vi "cloneAndCompare.vi"(9 "shapes":refnum<class "pShape.lvclass">[](array[class]), 10 "shapesCopy":refnum<class "pShape.lvclass">[](array[class])) -> ()   [LabVIEW 2017, in "PrototypePatternDemo.lvclass"]
uses:
  PrototypePatternDemo.lvclass
  Shape Class/pShape.lvclass
  ConsoleOut/Print Options.ctl
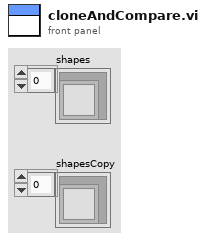
[diagram p1: front panel]
types:
  T1 = typedef "Print Options.ctl" = enum16{"Create", "Get Reference", "Print", "Print Header", "Close"}
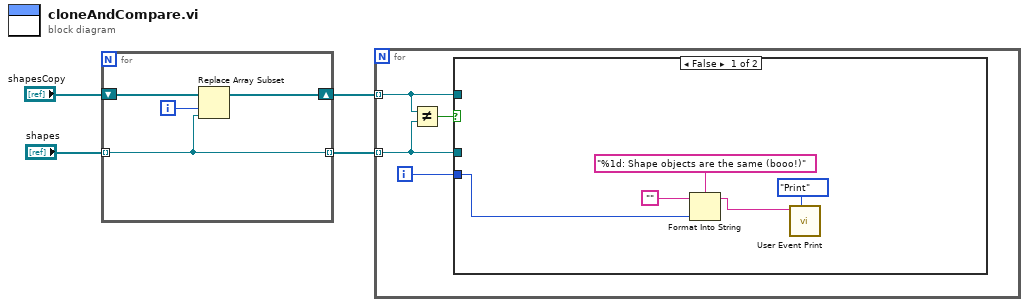
[diagram p0: block diagram]
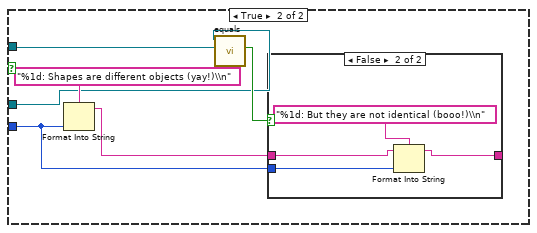
[diagram p2: hidden frame]
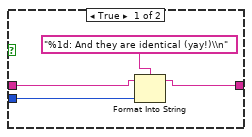
[diagram p3: hidden frame]
diagram:
  n1 = for {
    shift-right: [w8] -> w1
    shift-left: "shapesCopy" -> [w7]
    tunnel: "shapes" -> [w6] mode=indexing
    tunnel: [w6] -> w2 mode=indexing
    i -> [w5]
    n2 = Replace Array Subset(array=w7, new element=w6, index=w5) -> (w8:refnum<class "pShape.lvclass">[])
  }
  n3 = for {
    tunnel: w2 -> [w10] mode=indexing
    tunnel: w1 -> [w9] mode=indexing
    i -> [w11]
    n4 = Not Equal?(x=w9, y=w10) -> (x != y?=w12:bool)
    n5 = case shown="False" w12 {
      tunnel: w11 -> [w16 w18]
      tunnel: w10 -> [_ w21]
      tunnel: w9 -> [_ w20]
      frame False {
        n6 = Format Into String(format string="%1d: Shape objects are the same (booo!)", initial string="", w16) -> (resulting string=w14:string)  [unwired: 1 in, 1 out]
        n7 = call "User Event Print.vi"("Options"=Print_Options."Print", "String to Print"=w14) -> ()  [unwired: 8 in, 2 out]
      }
      frame True {
        n8 = Format Into String(format string="%1d: Shapes are different objects (yay!)\\n", w18) -> (resulting string=w19:string)  [unwired: 2 in, 1 out]
        n9 = call-dynamic "equals.vi"("object 2"=w20, "pShape in"=w21) -> ("equal?"=w22:bool)  [unwired: 7 in, 2 out]
        n10 = case shown="False" w22 {
          tunnel: w18 -> [w26 w30]
          tunnel: [w25 w29] -> _
          tunnel: w19 -> [w24 w28]
          frame True {
            n11 = Format Into String(format string="%1d: And they are identical (yay!)\\n", initial string=w24, w26) -> (resulting string=w25:string)  [unwired: 1 in, 1 out]
          }
          frame False {
            n12 = Format Into String(format string="%1d: But they are not identical (booo!)\\n", initial string=w28, w30) -> (resulting string=w29:string)  [unwired: 1 in, 1 out]
          }
        }
      }
    }
  }
